vi "SwapInstanceVIUnusedName2 6.vi"(4 "Comment (Create only)":string, 6 "Operation (Read or Create)":T1, 7 "Section":string, 8 "error in (no error)":errorcluster, 9 "Value":string, 10 "Key":string, 11 "Ini Path in":path) -> (0 "error out":errorcluster, 1 "Found?":bool, 2 "Value out":string, 3 "Ini Path out":path)   [LabVIEW 2018]
uses:
  lib/Cfg/Cfg.lvlib
  <vilib>/ErrorRing/Error Ring.xnode
  <vilib>/Utility/error.llb/Error Cluster From Error Code.vi
  lib/Cfg/Operation.ctl
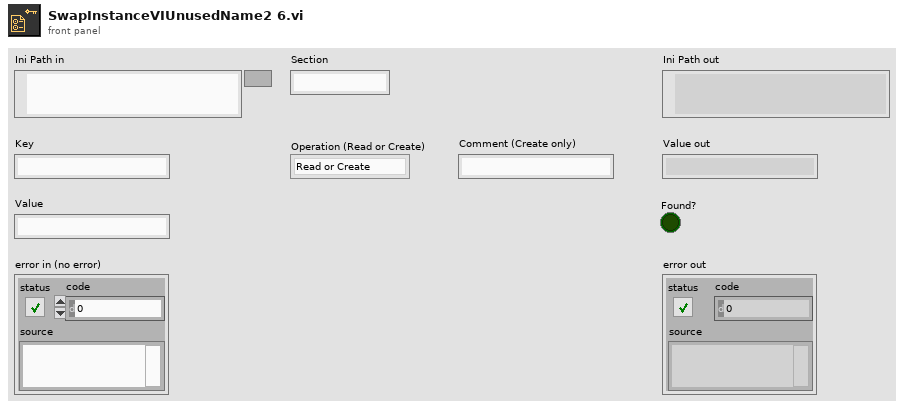
[diagram p1: front panel]
types:
  T1 = typedef "Cfg.lvlib/Operation.ctl" = enum8{"Read or Create", "Read", "Write"}
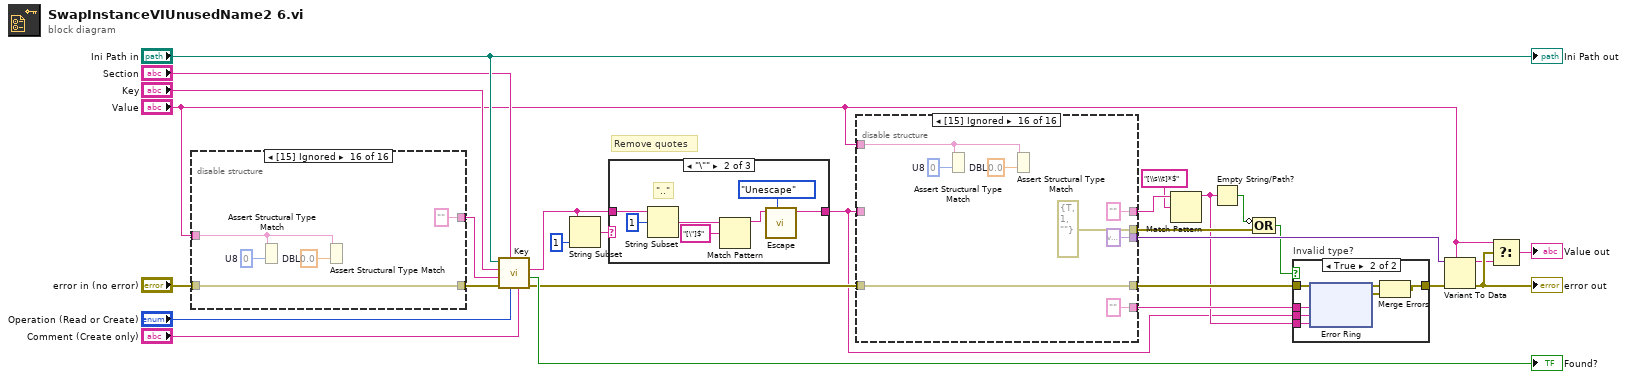
[diagram p0: block diagram]
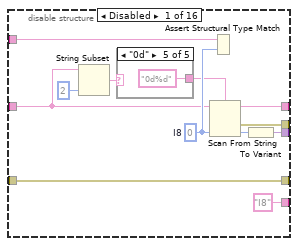
[diagram p2: hidden frame]
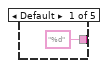
[diagram p3: hidden frame]
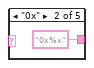
[diagram p4: hidden frame]
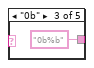
[diagram p5: hidden frame]
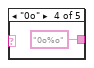
[diagram p6: hidden frame]
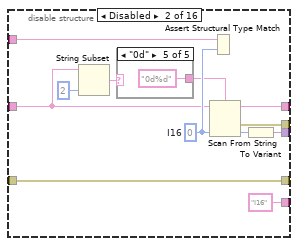
[diagram p7: hidden frame]
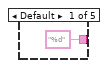
[diagram p8: hidden frame]
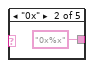
[diagram p9: hidden frame]
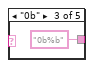
[diagram p10: hidden frame]
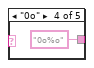
[diagram p11: hidden frame]
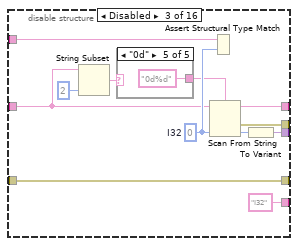
[diagram p12: hidden frame]
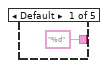
[diagram p13: hidden frame]
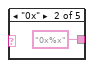
[diagram p14: hidden frame]
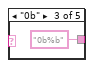
[diagram p15: hidden frame]
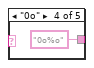
[diagram p16: hidden frame]
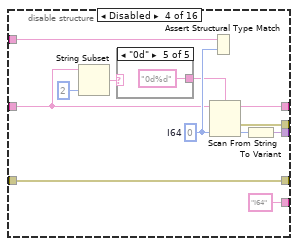
[diagram p17: hidden frame]
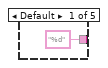
[diagram p18: hidden frame]
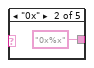
[diagram p19: hidden frame]
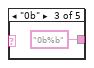
[diagram p20: hidden frame]
diagram:
  # "Remove quotes"
  n1 = disable-structure shown="[15] Ignored" {
    disable-tunnel: [w33 w38 w43 w48 w53 w58 w63 w68 w73 w78 w83 w88 w97 w104 w116 w121] -> w22
    disable-tunnel: "error in (no error)" -> [w33 w38 w43 w48 w53 w58 w63 w68 w73 w78 w83 w88 w97 w104 w116 w121]
    disable-tunnel: "Value" -> [w31 w36 w41 w46 w51 w56 w61 w66 w71 w76 w81 w87 w89 w98 w110 w117]
    disable-tunnel: [w30 w35 w40 w45 w50 w55 w60 w65 w70 w75 w80 w86 w91 w103 w115 ""] -> w20
    frame Disabled {
      w32 = i8 0  # I8
      n2 = Assert Structural Type Match(0:w32, 1:w31) -> ()
      n3 = Format Into String(format string="%d", w31) -> (resulting string=w30:string)  [unwired: 2 in, 1 out]
    }
    frame Disabled {
      w37 = i16 0  # I16
      n4 = Assert Structural Type Match(0:w37, 1:w36) -> ()
      n5 = Format Into String(format string="%d", w36) -> (resulting string=w35:string)  [unwired: 2 in, 1 out]
    }
    frame Disabled {
      w42 = 0  # I32
      n6 = Assert Structural Type Match(0:w42, 1:w41) -> ()
      n7 = Format Into String(format string="%d", w41) -> (resulting string=w40:string)  [unwired: 2 in, 1 out]
    }
    frame Disabled {
      w47 = i64 0  # I64
      n8 = Assert Structural Type Match(0:w47, 1:w46) -> ()
      n9 = Format Into String(format string="%d", w46) -> (resulting string=w45:string)  [unwired: 2 in, 1 out]
    }
    frame Disabled {
      w52 = u8 0  # U8
      n10 = Assert Structural Type Match(0:w52, 1:w51) -> ()
      n11 = Format Into String(format string="%u", w51) -> (resulting string=w50:string)  [unwired: 2 in, 1 out]
    }
    frame Disabled {
      w57 = u16 0  # U16
      n12 = Assert Structural Type Match(0:w57, 1:w56) -> ()
      n13 = Format Into String(format string="%u", w56) -> (resulting string=w55:string)  [unwired: 2 in, 1 out]
    }
    frame Disabled {
      w62 = u32 0  # U32
      n14 = Assert Structural Type Match(0:w62, 1:w61) -> ()
      n15 = Format Into String(format string="%u", w61) -> (resulting string=w60:string)  [unwired: 2 in, 1 out]
    }
    frame Disabled {
      w67 = u64 0  # U64
      n16 = Assert Structural Type Match(0:w67, 1:w66) -> ()
      n17 = Format Into String(format string="%u", w66) -> (resulting string=w65:string)  [unwired: 2 in, 1 out]
    }
    frame Disabled {
      w72 = sgl 0.0  # SGL
      n18 = Assert Structural Type Match(0:w72, 1:w71) -> ()
      n19 = Format Into String(format string="%#.12g", w71) -> (resulting string=w70:string)  [unwired: 2 in, 1 out]
    }
    frame Disabled {
      w77 = 0.0  # DBL
      n20 = Assert Structural Type Match(0:w77, 1:w76) -> ()
      n21 = Format Into String(format string="%#.12g", w76) -> (resulting string=w75:string)  [unwired: 2 in, 1 out]
    }
    frame Disabled {
      w82 = ext 0.0  # EXT
      n22 = Assert Structural Type Match(0:w82, 1:w81) -> ()
      n23 = Format Into String(format string="%#.12g", w81) -> (resulting string=w80:string)  [unwired: 2 in, 1 out]
    }
    frame Disabled {
      n24 = Assert Structural Type Match(0:FALSE, 1:w87) -> ()
      n25 = Format Into String(format string="%s", w87) -> (resulting string=w86:string)  [unwired: 2 in, 1 out]
    }
    frame Disabled {
      # "enum"
      n26 = Format Into String(format string="%u", w89) -> ()  [unwired: 2 in, 2 out]
      n27 = Format Into String(format string="%s", w89) -> (resulting string=w92:string)  [unwired: 2 in, 1 out]
      n28 = call "Escape.vi"("Action"=enum8{"Escape", "Unescape"}."Escape", "String in"=w92) -> ("String out"=w93:string)  [unwired: 8 in, 1 out]
      n29 = Format Into String(format string="\"%s\"", w93) -> (resulting string=w91:string)  [unwired: 2 in, 1 out]
    }
    frame Enabled {
      n30 = Assert Structural Type Match(0:"", 1:w98) -> ()
      n31 = call "Escape.vi"("Action"=enum8{"Escape", "Unescape"}."Escape", "String in"=w98) -> ("String out"=w100:string)  [unwired: 8 in, 1 out]
      n32 = Format Into String(format string="\"%s\"", w100) -> (resulting string=w103:string)  [unwired: 2 in, 1 out]
    }
    frame Disabled {
      n33 = Assert Structural Type Match(0:path "", 1:w110) -> ()
      n34 = Path To String(path=w110) -> (string=w109:string)
      n35 = Search and Replace String(replace all?=TRUE ("replace all? (F)"), input string=w109, search string="\\", replace string="/" ("replace string (\"\")")) -> (result string=w108:string)  [unwired: 4 in, 3 out]
      n36 = call "Escape.vi"("Action"=enum8{"Escape", "Unescape"}."Escape", "String in"=w108) -> ("String out"=w113:string)  [unwired: 8 in, 1 out]
      n37 = Format Into String(format string="\"%s\"", w113) -> (resulting string=w115:string)  [unwired: 2 in, 1 out]
    }
    frame Disabled {
      w118 = 0.0  # DBL
      w119 = u8 0  # U8
      n38 = Assert Structural Type Match(0:w119, 1:w117) -> ()
      n39 = Assert Structural Type Match(0:w118, 1:w117) -> ()
    }
  }
  n40 = call "Key.vi"("Comment (Create only)"="Comment (Create only)", "Operation (Read or Create)"="Operation (Read or Create)", "Section"="Section", "error in (no error)"=w22, "Value"=w20, "Key"="Key", "Ini Path in"="Ini Path in") -> ("error out"=w19:errorcluster, "Found?"=→"Found?":bool, "Value out"=w10:string)  [unwired: 1 in, 1 out]
  n41 = String Subset(string=w10, length (rest)=1 ("length (rest)")) -> (substring=w11:string)  [unwired: 1 in]
  n42 = case shown="\"\\\"\"" w11 {
    tunnel: w10 -> [w122 w128 w135]
    tunnel: [w122 w126 w133] -> w1
    frame Default {
    }
    frame "\"" {
      # "\"..\""
      n43 = String Subset(string=w128, offset (0)=1) -> (substring=w125:string)  [unwired: 1 in]
      n44 = Match Pattern(string=w125, regular expression="[\"]$") -> (before substring=w123:string)  [unwired: 1 in, 3 out]
      n45 = call "Escape.vi"("Action"=enum8{"Escape", "Unescape"}."Unescape", "String in"=w123) -> ("String out"=w126:string)  [unwired: 8 in, 1 out]
    }
    frame "'" {
      # "'..'"
      n46 = String Subset(string=w135, offset (0)=1) -> (substring=w132:string)  [unwired: 1 in]
      n47 = Match Pattern(string=w132, regular expression="[']$") -> (before substring=w130:string)  [unwired: 1 in, 3 out]
      n48 = call "Escape.vi"("Action"=enum8{"Escape", "Unescape"}."Unescape", "String in"=w130) -> ("String out"=w133:string)  [unwired: 8 in, 1 out]
    }
  }
  n49 = disable-structure shown="[15] Ignored" {
    disable-tunnel: [w148 w165 w182 w199 w216 w233 w250 w267 w282 w292 w302 w311 w328 w340 w358 w366] -> w18
    disable-tunnel: w19 -> [w148 w165 w182 w199 w216 w233 w250 w267 w282 w292 w302 w311 w328 w340 w358 w366]
    disable-tunnel: "Value" -> [w147 w164 w181 w198 w215 w232 w249 w266 w281 w291 w301 w310 w318 w339 w357 w361]
    disable-tunnel: w1 -> [w145 w162 w179 w196 w213 w230 w247 w264 w279 w289 w299 w306 w324 w334 w348 _]
    disable-tunnel: [w141 w158 w175 w192 w209 w226 w243 w260 w277 w287 w297 w304 w319 "" "" ""] -> w9
    disable-tunnel: [w140 w157 w174 w191 w208 w225 w242 w259 w276 w286 w296 errorcluster {"status"=FALSE, "code"=0, "source"=""} ("error IO") w322 errorcluster {"status"=FALSE, "code"=0, "source"=""} ("error IO") errorcluster {"status"=FALSE, "code"=0, "source"=""} ("error IO") errorcluster {"status"=TRUE, "code"=1, "source"=""} ("error IO")] -> w6
    disable-tunnel: [w138 w155 w172 w189 w206 w223 w240 w257 w274 w284 w294 w308 w320 w337 w355 variant ("Variant")] -> w13
    disable-tunnel: ["I8" "I16" "I32" "I64" "U8" "U16" "U32" "U64" "SGL" "DBL" "EXT" "Boolean" w327 "String" "Path" ""] -> w3
    frame Disabled {
      w146 = i8 0  # I8
      n50 = String Subset(string=w145, length (rest)=2 ("length (rest)")) -> (substring=w143:string)  [unwired: 1 in]
      n51 = case shown="\"0d\"" w143 {
        tunnel: ["%d" "0x%x" "0b%b" "0o%o" "0d%d"] -> w142
        frame Default {
        }
        frame "0x" {
        }
        frame "0b" {
        }
        frame "0o" {
        }
        frame "0d" {
        }
      }
      n52 = Assert Structural Type Match(0:w146, 1:w147) -> ()
      n53 = Scan From String(format string=w142, input string=w145, default 1=w146) -> (remaining string=w141:string, error out=w140:errorcluster, output 1=w139:i8)  [unwired: 2 in, 1 out]
      n54 = To Variant(anything=w139) -> (Variant=w138:variant)
    }
    frame Disabled {
      w163 = i16 0  # I16
      n55 = String Subset(string=w162, length (rest)=2 ("length (rest)")) -> (substring=w160:string)  [unwired: 1 in]
      n56 = case shown="\"0d\"" w160 {
        tunnel: ["%d" "0x%x" "0b%b" "0o%o" "0d%d"] -> w159
        frame Default {
        }
        frame "0x" {
        }
        frame "0b" {
        }
        frame "0o" {
        }
        frame "0d" {
        }
      }
      n57 = Assert Structural Type Match(0:w163, 1:w164) -> ()
      n58 = Scan From String(format string=w159, input string=w162, default 1=w163) -> (remaining string=w158:string, error out=w157:errorcluster, output 1=w156:i16)  [unwired: 2 in, 1 out]
      n59 = To Variant(anything=w156) -> (Variant=w155:variant)
    }
    frame Disabled {
      w180 = 0  # I32
      n60 = String Subset(string=w179, length (rest)=2 ("length (rest)")) -> (substring=w177:string)  [unwired: 1 in]
      n61 = case shown="\"0d\"" w177 {
        tunnel: ["%d" "0x%x" "0b%b" "0o%o" "0d%d"] -> w176
        frame Default {
        }
        frame "0x" {
        }
        frame "0b" {
        }
        frame "0o" {
        }
        frame "0d" {
        }
      }
      n62 = Assert Structural Type Match(0:w180, 1:w181) -> ()
      n63 = Scan From String(format string=w176, input string=w179, default 1=w180) -> (remaining string=w175:string, error out=w174:errorcluster, output 1=w173:i32)  [unwired: 2 in, 1 out]
      n64 = To Variant(anything=w173) -> (Variant=w172:variant)
    }
    frame Disabled {
      w197 = i64 0  # I64
      n65 = String Subset(string=w196, length (rest)=2 ("length (rest)")) -> (substring=w194:string)  [unwired: 1 in]
      n66 = case shown="\"0d\"" w194 {
        tunnel: ["%d" "0x%x" "0b%b" "0o%o" "0d%d"] -> w193
        frame Default {
        }
        frame "0x" {
        }
        frame "0b" {
        }
        frame "0o" {
        }
        frame "0d" {
        }
      }
      n67 = Assert Structural Type Match(0:w197, 1:w198) -> ()
      n68 = Scan From String(format string=w193, input string=w196, default 1=w197) -> (remaining string=w192:string, error out=w191:errorcluster, output 1=w190:i64)  [unwired: 2 in, 1 out]
      n69 = To Variant(anything=w190) -> (Variant=w189:variant)
    }
    frame Disabled {
      w214 = u8 0  # U8
      n70 = String Subset(string=w213, length (rest)=2 ("length (rest)")) -> (substring=w211:string)  [unwired: 1 in]
      n71 = case shown="Default" w211 {
        tunnel: ["%u" "0x%x" "0b%b" "0o%o" "0d%u"] -> w210
        frame Default {
        }
        frame "0x" {
        }
        frame "0b" {
        }
        frame "0o" {
        }
        frame "0d" {
        }
      }
      n72 = Assert Structural Type Match(0:w214, 1:w215) -> ()
      n73 = Scan From String(format string=w210, input string=w213, default 1=w214) -> (remaining string=w209:string, error out=w208:errorcluster, output 1=w207:u8)  [unwired: 2 in, 1 out]
      n74 = To Variant(anything=w207) -> (Variant=w206:variant)
    }
    frame Disabled {
      w231 = u16 0  # U16
      n75 = String Subset(string=w230, length (rest)=2 ("length (rest)")) -> (substring=w228:string)  [unwired: 1 in]
      n76 = case shown="Default" w228 {
        tunnel: ["%u" "0x%x" "0b%b" "0o%o" "0d%u"] -> w227
        frame Default {
        }
        frame "0x" {
        }
        frame "0b" {
        }
        frame "0o" {
        }
        frame "0d" {
        }
      }
      n77 = Assert Structural Type Match(0:w231, 1:w232) -> ()
      n78 = Scan From String(format string=w227, input string=w230, default 1=w231) -> (remaining string=w226:string, error out=w225:errorcluster, output 1=w224:u16)  [unwired: 2 in, 1 out]
      n79 = To Variant(anything=w224) -> (Variant=w223:variant)
    }
    frame Disabled {
      w248 = u32 0  # U32
      n80 = String Subset(string=w247, length (rest)=2 ("length (rest)")) -> (substring=w245:string)  [unwired: 1 in]
      n81 = case shown="Default" w245 {
        tunnel: ["%u" "0x%x" "0b%b" "0o%o" "0d%u"] -> w244
        frame Default {
        }
        frame "0x" {
        }
        frame "0b" {
        }
        frame "0o" {
        }
        frame "0d" {
        }
      }
      n82 = Assert Structural Type Match(0:w248, 1:w249) -> ()
      n83 = Scan From String(format string=w244, input string=w247, default 1=w248) -> (remaining string=w243:string, error out=w242:errorcluster, output 1=w241:u32)  [unwired: 2 in, 1 out]
      n84 = To Variant(anything=w241) -> (Variant=w240:variant)
    }
    frame Disabled {
      w265 = u64 0  # U64
      n85 = String Subset(string=w264, length (rest)=2 ("length (rest)")) -> (substring=w262:string)  [unwired: 1 in]
      n86 = case shown="Default" w262 {
        tunnel: ["%u" "0x%x" "0b%b" "0o%o" "0d%u"] -> w261
        frame Default {
        }
        frame "0x" {
        }
        frame "0b" {
        }
        frame "0o" {
        }
        frame "0d" {
        }
      }
      n87 = Assert Structural Type Match(0:w265, 1:w266) -> ()
      n88 = Scan From String(format string=w261, input string=w264, default 1=w265) -> (remaining string=w260:string, error out=w259:errorcluster, output 1=w258:u64)  [unwired: 2 in, 1 out]
      n89 = To Variant(anything=w258) -> (Variant=w257:variant)
    }
    frame Disabled {
      w280 = sgl 0.0  # SGL
      n90 = Assert Structural Type Match(0:w280, 1:w281) -> ()
      n91 = Scan From String(format string="%f", input string=w279, default 1=w280) -> (remaining string=w277:string, error out=w276:errorcluster, output 1=w275:sgl)  [unwired: 2 in, 1 out]
      n92 = To Variant(anything=w275) -> (Variant=w274:variant)
    }
    frame Disabled {
      w290 = 0.0  # DBL
      n93 = Assert Structural Type Match(0:w290, 1:w291) -> ()
      n94 = Scan From String(format string="%f", input string=w289, default 1=w290) -> (remaining string=w287:string, error out=w286:errorcluster, output 1=w285:dbl)  [unwired: 2 in, 1 out]
      n95 = To Variant(anything=w285) -> (Variant=w284:variant)
    }
    frame Disabled {
      w300 = ext 0.0  # EXT
      n96 = Assert Structural Type Match(0:w300, 1:w301) -> ()
      n97 = Scan From String(format string="%f", input string=w299, default 1=w300) -> (remaining string=w297:string, error out=w296:errorcluster, output 1=w295:ext)  [unwired: 2 in, 1 out]
      n98 = To Variant(anything=w295) -> (Variant=w294:variant)
    }
    frame Disabled {
      n99 = case shown="Default" w306 {
        selector: w306 -> [w312 _ _]
        tunnel: [FALSE TRUE FALSE] -> w305
        tunnel: [w312 _ _] -> w304
        frame Default {
        }
        frame "1", "True" {
        }
        frame "0", "False" {
        }
      }
      n100 = Assert Structural Type Match(0:FALSE, 1:w310) -> ()
      n101 = To Variant(anything=w305) -> (Variant=w308:variant)
    }
    frame Disabled {
      # "enum"
      n102 = Format Into String(format string="%u", w318) -> ()  [unwired: 2 in, 2 out]
      n103 = Type Cast(x=w318) -> (*(type *) &x=w317:string)  [unwired: 1 in]
      n104 = String Length(string=w317) -> (length=w316:i32)
      n105 = Format Into String(format string="%s", w318) -> ()  [unwired: 2 in, 2 out]
      n106 = case shown="5..8" w316 {
        tunnel: ["Enum U8" "Enum U16" "Enum U32" "Enum U64"] -> w327
        frame 1, Default {
        }
        frame 2 {
        }
        frame 3, 4 {
        }
        frame 5..8 {
        }
      }
      n107 = Scan From String(format string="%s", input string=w324, default 1=w318) -> (remaining string=w319:string, error out=w322:errorcluster, output 1=w321:string)  [unwired: 2 in, 1 out]
      n108 = To Variant(anything=w321) -> (Variant=w320:variant)
    }
    frame Enabled {
      n109 = Assert Structural Type Match(0:"", 1:w339) -> ()
      n110 = To Variant(anything=w334) -> (Variant=w337:variant)
    }
    frame Disabled {
      w343 = 1 ("offset (0)")
      n111 = Array of Strings to Path(0:string[] ["a", "a"] ("array of strings"), 1:TRUE ("relative")) -> (2:w344:path)
      n112 = Path To String(path=w344) -> (string=w342:string)
      n113 = String Subset(string=w342, offset (0)=w343, length (rest)=w343) -> (substring=w341:string)
      n114 = Search and Replace String(replace all?=TRUE ("replace all? (F)"), input string=w348, search string="/", replace string=w341) -> (result string=w349:string)  [unwired: 4 in, 3 out]
      n115 = String To Path(string=w349) -> (path=w347:path)
      n116 = Assert Structural Type Match(0:path "", 1:w357) -> ()
      n117 = To Variant(anything=w347) -> (Variant=w355:variant)
    }
    frame Disabled {
      w363 = 0.0  # DBL
      w362 = u8 0  # U8
      n118 = Assert Structural Type Match(0:w362, 1:w361) -> ()
      n119 = Assert Structural Type Match(0:w363, 1:w361) -> ()
    }
  }
  n120 = Match Pattern(string=w9, regular expression="[\\s\\t]*$") -> (before substring=w2:string)  [unwired: 1 in, 3 out]
  n121 = Empty String/Path?(string/path=w2) -> (empty?=w7:bool)
  n122 = Compound Arithmetic op=OR(invert w7, w6) -> (w4:bool)
  n123 = case "Invalid type?" shown="True" w4 {
    tunnel: w18 -> [w367 w373]
    tunnel: [w367 w372] -> w5
    tunnel: w3 -> [_ w370]
    tunnel: w2 -> [_ w369]
    tunnel: w1 -> [_ w368]
    frame False {
    }
    frame True {
      n124 = xnode "Error Ring"("parameter 0"=w370, "parameter 1"=w368, "parameter 2"=w369) -> ("error out"=w371:errorcluster)
      n125 = Merge Errors(w373, w371) -> (w372:errorcluster)
    }
  }
  n126 = Variant To Data(error in=w5, type="Value", Variant=w13) -> (data=w15:string, error out=w16:errorcluster)
  "error out" <- w16
  n127 = Select(t="Value", s=w16, f=w15) -> (s? t:f=→"Value out":string)
  "Ini Path out" <- "Ini Path in"
